vi "Unit Test.vi"() -> ()   [LabVIEW 2019, in "LED.lvlib"]
uses:
  LED.lvlib
  User Event/Controls/UE Abort Action.ctl
panel:
  in  "Open":bool
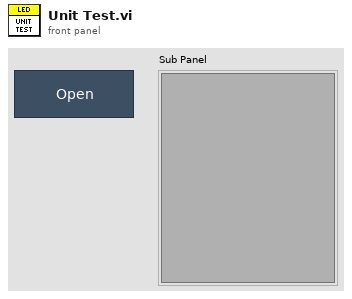
[diagram p1: front panel]
types:
  T1 = typedef "UE Abort Action.ctl" = enum16{"Create", "Get", "Destroy"}
  T2 = typedef "LED.lvlib/SEQ Data.ctl" = cluster{"Initialize Sucess?":bool, "BL2 Regulator":dbl, "BL1 Regulator":dbl, "Blood Sensor 1":dbl, "Blood Sensor 2":dbl, "Air Pressure Sensor":dbl, "Force Snesor 1":u32, "Force Snesor 2":u32, "VI Refnum":refnum<vi>}
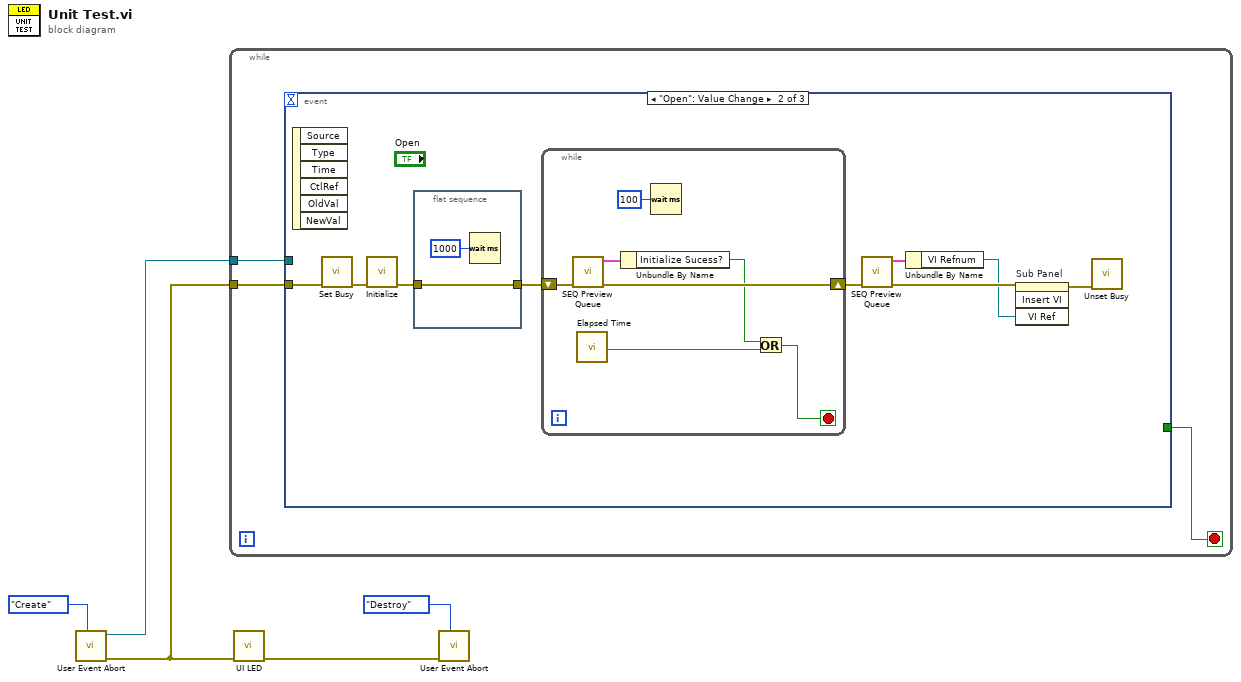
[diagram p0: block diagram]
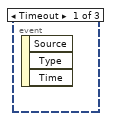
[diagram p2: hidden frame]
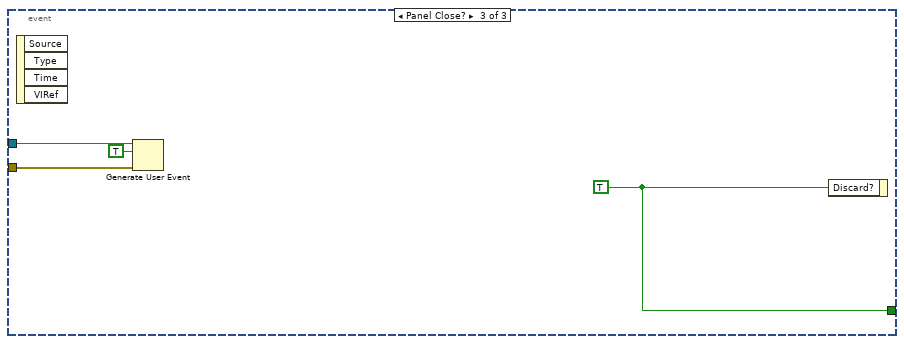
[diagram p3: hidden frame]
diagram:
  n1 = call "User Event Abort.vi"("Action"=UE_Abort_Action."Create") -> ("Error Out"=w1:errorcluster, "User Event Out"=w2:refnum<user-event>)  [unwired: 9 in]
  n2 = while {
    tunnel: w2 -> [w8]
    tunnel: w1 -> [w6]
    stop <- w7 stop-if-true
    n3 = event shown="[1] \"Open\": Value Change" {
      selector: _ -> [_ _ _]
      dyn-events: _ -> [_ _ _]
      timeout: _ -> [_ _ _]
      tunnel: w8 -> [_ _ w29]
      tunnel: [_ _ w30] -> w7
      tunnel: w6 -> [_ w17 w28]
      event Timeout {
        n4 = event-data() -> ()  [unwired: 1 in, 3 out]
      }
      event "Open": Value Change {
        n5 = event-data() -> ()  [unwired: 1 in, 6 out]
        n6 = call <vilib>:"Set Busy.vi"("error in (no error)"=w17) -> ("error out"=w16:errorcluster)  [unwired: 9 in, 1 out]
        n7 = call "Initialize.vi"("Error In"=w16) -> ("Error Out"=w15:errorcluster)  [unwired: 10 in]
        n8 = flat-sequence {
          tunnel: w15 -> [w25]
          tunnel: [w25] -> w14
          frame #0 {
            n9 = Wait (ms)(milliseconds to wait=u32 1000) -> ()  [unwired: 1 out]
          }
        }
        n10 = while {
          shift-right: [w22] -> w13
          shift-left: w14 -> [w24]
          stop <- w18 stop-if-true
          n11 = call "SEQ Preview Queue.vi"("error in"=w24) -> ("error out"=w22:errorcluster, "SEQ Data"=w21:T2)  [unwired: 9 in]
          n12 = call "Elapsed Time"() -> ("Time has Elapsed"=w19:bool)  [unwired: 12 in, 7 out]
          n13 = Unbundle By Name(w21) -> ("Initialize Sucess?"=w20:bool)
          n14 = Wait (ms)(milliseconds to wait=u32 100) -> ()  [unwired: 1 out]
          n15 = Or(x=w20, y=w19) -> (x .or. y?=w18:bool)
        }
        n16 = call "SEQ Preview Queue.vi"("error in"=w13) -> ("error out"=w11:errorcluster, "SEQ Data"=w12:T2)  [unwired: 9 in]
        n17 = Unbundle By Name(w12) -> ("VI Refnum"=w9:refnum<vi>)
        n18 = invoke on="Sub Panel" class="SubPnl" method="Insert VI"(error in=w11, "VI Ref"=w9) -> (error out=w10:errorcluster)  [unwired: 2 in, 3 out]
        n19 = call <vilib>:"Unset Busy.vi"("error in (no error)"=w10) -> ()  [unwired: 10 in, 1 out]
      }
      event Panel Close? {
        w30 = TRUE ("Discard?")
        n20 = event-data() -> ()  [unwired: 1 in, 4 out]
        n21 = Generate User Event(user event=w29, event data cluster=TRUE ("event data"), error in=w28) -> ()  [unwired: 1 in, 2 out]
        n22 = event-data("Discard?"=w30) -> ()  [unwired: 1 in, 1 out]
      }
    }
  }
  n23 = call "UI LED.vi"("error in"=w1) -> ("error out"=w5:errorcluster)  [unwired: 10 in]
  n24 = call "User Event Abort.vi"("Action"=UE_Abort_Action."Destroy", "Error In"=w5) -> ()  [unwired: 8 in, 2 out]
